vi "test Merge Import Aliases.vi"(8 "error in (no error)":errorcluster, 11 "TestCase in":refnum<class "Routing and Faulting Import Unit Tests.lvclass">) -> (0 "error out":errorcluster, 3 "TestCase out":refnum<class "Routing and Faulting Import Unit Tests.lvclass">)   [LabVIEW 2020, in "Routing and Faulting Import Unit Tests.lvclass"]
uses:
  Routing and Faulting Import Unit Tests.lvclass
  Shared/Alias Mapping.ctl
  Shared/Alias Endpoint.ctl
  Routing and Faulting Import Unit Tests.lvclass/Routing and Faulting Import Unit Tests.ctl
  <userlib>/_OpenG.lib/file/file.llb/Append Path to Root if Relative - Scalar__ogtk.vi
  <vilib>/addons/_JKI Toolkits/VI Tester/TestCase.llb/TestCase.lvclass
  <vilib>/NI/VeriStand Custom Device Testing Tools/VeriStandTestUtilities/VeriStandTestUtilities.lvlib
  Scripting/Routing and Faulting Scripting.lvlib
  Shared/Routing and Faulting Shared.lvlib
  C:/Program Files (x86)/National Instruments/LabVIEW 2020/vi.lib/addons/_JKI Toolkits/VI Tester/TestCase.llb/TestCase.lvclass
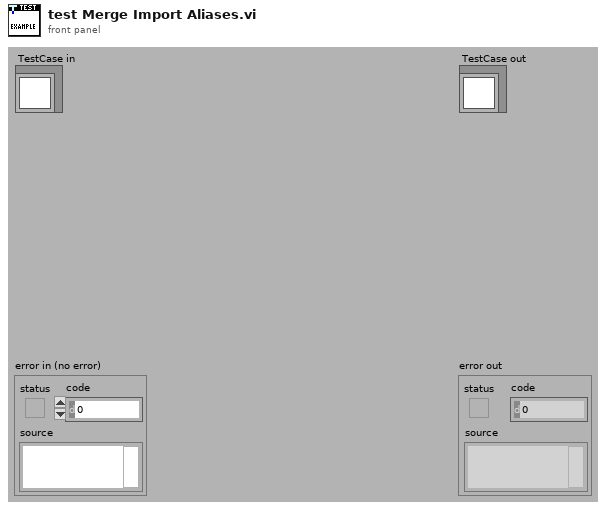
[diagram p1: front panel]
types:
  T1 = typedef "Routing and Faulting Shared.lvlib/Alias Mapping.ctl" = cluster{"Alias":string, "Endpoint":T2}
  T2 = typedef "Routing and Faulting Shared.lvlib/Alias Endpoint.ctl" = cluster{"Module Path":string, "Endpoint":string}
  T3 = typedef "Custom Device API.lvlib/Custom Device Item Ref.ctl" = u64
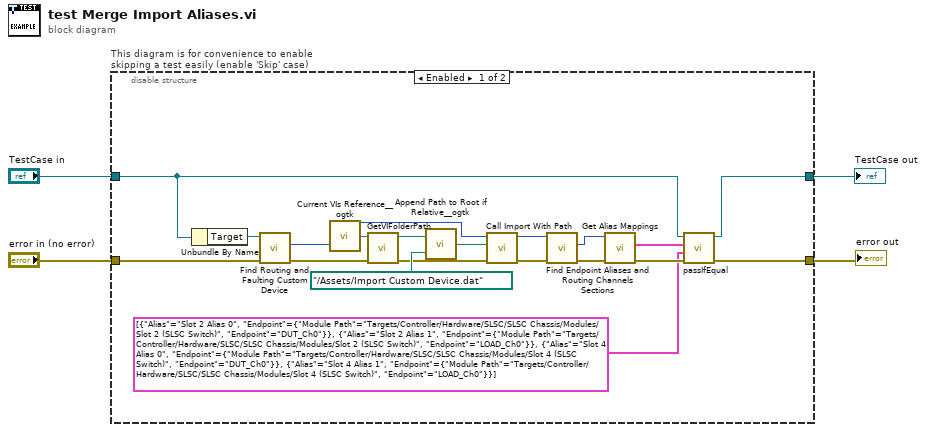
[diagram p0: block diagram]
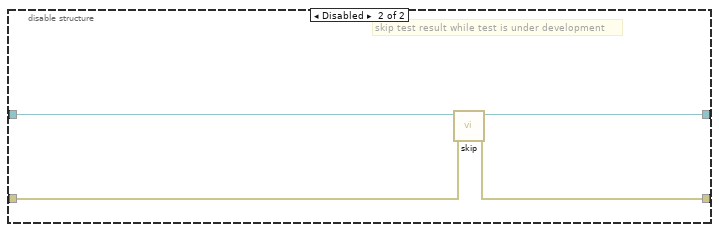
[diagram p2: hidden frame]
diagram:
  n1 = disable-structure "This diagram is for convenience to enable skipping a test easily (enable 'Skip' case)" shown="Enabled" {
    disable-tunnel: "TestCase in" -> [w11 w27]
    disable-tunnel: [w10 w25] -> w1
    disable-tunnel: [w9 w26] -> w3
    disable-tunnel: "error in (no error)" -> [w16 w24]
    frame Enabled {
      n2 = Unbundle By Name(w11) -> ("Target"=w17:refnum<k24>)
      n3 = call "Find Routing and Faulting Custom Device.vi"("error in"=w16, "target in"=w17) -> ("error out"=w18:errorcluster, "routing and faulting custom device"=w6:T3)  [unwired: 7 in, 1 out]
      n4 = call <userlib>:"Current VIs Reference__ogtk.vi"() -> ("Current VI's reference"=w23:refnum<vi>)  [unwired: 5 in]
      n5 = call <vilib>:"GetVIFolderPath.vi"("error in (no error)"=w18, "VI Reference in"=w23) -> ("error out"=w20:errorcluster, "VI Folder Path out"=w22:path)  [unwired: 8 in]
      n6 = call-poly <userlib>:"Append Path to Root if Relative__ogtk.vi"("Absolute or Relative Path"=path "../Assets/Import Custom Device.dat", "Root Path"=w22) -> ("Absolute or Appended Path"=w7:path)
      n7 = call "Call Import With Path.vi"("error in (no error)"=w20, "Path"=w7, "Routing and Faulting Custom Device Ref in"=w6) -> ("error out"=w19:errorcluster, "Routing and Faulting Custom Device Ref out"=w5:T3)  [unwired: 7 in]
      n8 = call "Find Endpoint Aliases and Routing Channels Sections.vi"("error in"=w19, "routing and faulting custom device in"=w5) -> ("error out"=w15:errorcluster, "endpoint aliases"=w14:T3)  [unwired: 6 in, 2 out]
      n9 = call "Get Alias Mappings.vi"("error in"=w15, "endpoint aliases in"=w14) -> ("error out"=w13:errorcluster, "alias mappings"=w12:T1[])  [unwired: 7 in, 1 out]
      n10 = call-dynamic "passIfEqual.vi"("error in (no error)"=w13, "y"=T1[] [{"Alias"="Slot 2 Alias 0", "Endpoint"={"Module Path"="Targets/Controller/Hardware/SLSC/SLSC Chassis/Modules/Slot 2 (SLSC Switch)", "Endpoint"="DUT_Ch0"}}, {"Alias"="Slot 2 Alias 1", "Endpoint"={"Module Path"="Targets/Controller/Hardware/SLSC/SLSC Chassis/Modules/Slot 2 (SLSC Switch)", "Endpoint"="LOAD_Ch0"}}, {"Alias"="Slot 4 Alias 0", "Endpoint"={"Module Path"="Targets/Controller/Hardware/SLSC/SLSC Chassis/Modules/Slot 4 (SLSC Switch)", "Endpoint"="DUT_Ch0"}}, {"Alias"="Slot 4 Alias 1", "Endpoint"={"Module Path"="Targets/Controller/Hardware/SLSC/SLSC Chassis/Modules/Slot 4 (SLSC Switch)", "Endpoint"="LOAD_Ch0"}}] ("Alias Mappings"), "x"=w12, "TestCase in"=w11) -> ("error out"=w9:errorcluster, "TestCase out"=w10:refnum<class "Routing and Faulting Import Unit Tests.lvclass">)  [unwired: 6 in]
    }
    frame Disabled {
      # "skip test result while test is under development"
      n11 = call <vilib>:"skip.vi"("error in (no error)"=w24, "TestCase in"=w27) -> ("error out"=w26:errorcluster, "TestCase out"=w25:refnum<class "Routing and Faulting Import Unit Tests.lvclass">)  [unwired: 8 in]
    }
  }
  "error out" <- w3
  "TestCase out" <- w1
